vi "Obtain ConfigureShape Event.vi"(8 "error in (no error)":errorcluster) -> (0 "error out":errorcluster, 3 "ShapeChanged Event":refnum<user-event>)   [LabVIEW 2017, in "LV Image Editor Framework.lvlib" / "Image Editor Handler.lvclass"]
uses:
  Image Editor Handler.lvclass
  Forms/Shape/Shape.lvclass
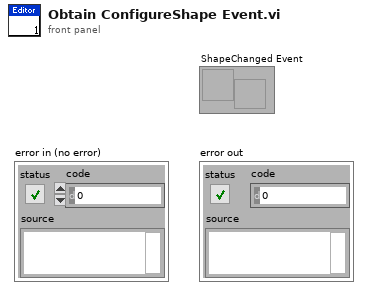
[diagram p1: front panel]
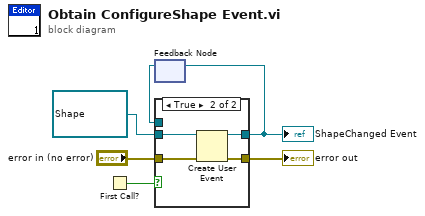
[diagram p0: block diagram]
diagram:
  n1 = First Call?() -> (First Call?: T/F=w4:bool)
  n2 = feedback #1() -> (w3:refnum<user-event>)  [unwired: 1 in]
  n3 = case shown="True" w4 {
    tunnel: "error in (no error)" -> [w7 w12]
    tunnel: [w8 w11] -> w2
    tunnel: w3 -> [w8 _]
    tunnel: refnum<data-value> refnum ("Shape in") -> [_ w10]
    tunnel: [w7 w9] -> w6
    frame False {
    }
    frame True {
      n4 = Create User Event(user event datatype=w10, error in=w12) -> (user event=w11:refnum<user-event>, error out=w9:errorcluster)
    }
  }
  "error out" <- w6
  "ShapeChanged Event" <- w2
  n5 = feedback-in #1(w2) -> ()
